vi "Test motor acceleration.vi"() -> ()   [LabVIEW 2016]
uses:
  <vilib>/Platform/TimedLoop/XDataNode/timing_clust.ctl
  <vilib>/Platform/TimedLoop/XDataNode/nitl_modes.ctl
  <vilib>/Platform/TimedLoop/XDataNode/wakeup.ctl
  <vilib>/Platform/TimedLoop/XDataNode/XDataNode.xnode
  <vilib>/Platform/TimedLoop/XDataNode/XDNodeRunTimeDep.lvlib
panel:
  in  "Disable motors":bool
  in  "Wheel velocity PID Right":T1={"P Gain"=0.8, "I Gain"=0.1, "D Gain"=0.002}
  in  "Wheel velocity PID Left":T1={"P Gain"=0.8, "I Gain"=0.1, "D Gain"=0.002}
  in  "Right motor speed rev/s":dbl
  in  "Left motor speed rev/s":dbl
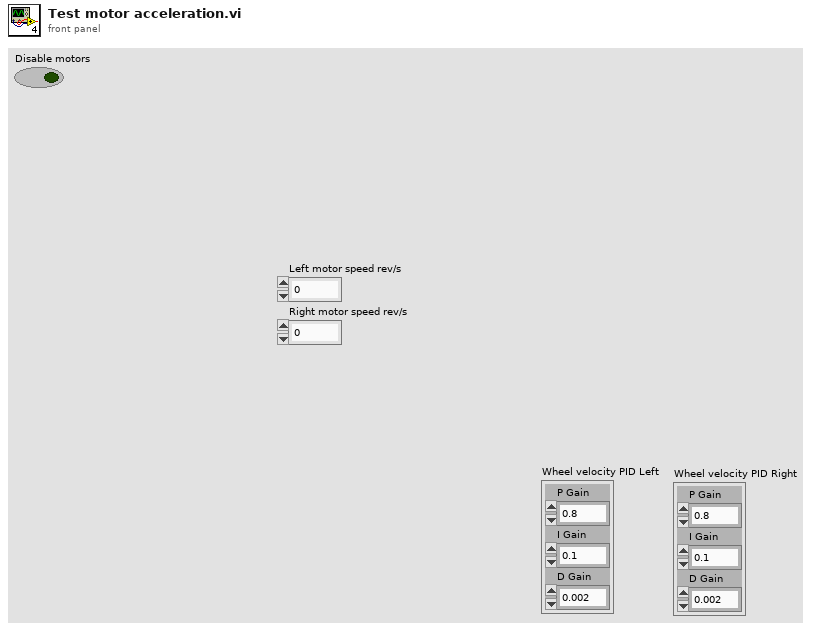
[diagram p1: front panel]
types:
  T1 = cluster{"P Gain":dbl, "I Gain":dbl, "D Gain":dbl}
  T2 = typedef "XDNodeRunTimeDep.lvlib/timing_clust.ctl" = cluster{"Expected End [f-1]":u64, "Actual End [f-1]":u64, "Finished Late? [f-1]":bool, "Expected End [i-1]":u64, "Actual End [i-1]":u64, "Finished Late? [i-1]":bool, "Expected Start [i]":u64, "Actual Start [i]":u64, "Expected Start [f]":u64, "Actual Start [f]":u64, "Source Name":string, "Structure Name":string, "Period":i64, "Deadline":i64, "Offset":i64, "Start":i64, "Priority":i32, "Timeout":i32, "Mode":T3, "Wakeup Reason":T4, "Error":errorcluster, "Source Type":string, "Secondary Source Type":string, "Global End Time":u64, "Global Start Time":u64, "Frame Duration":u64, "Iteration Duration":u64, "Assigned CPU":i32, "I/O Scan Engine Mode":u32}
  T3 = typedef "XDNodeRunTimeDep.lvlib/nitl_modes.ctl" = enum32{"No Change", "Process missed periods, maintain original phase", "Discard missed periods, maintain original phase", "Process missed periods, ignore original phase", "Discard missed periods, ignore original phase"}
  T4 = typedef "XDNodeRunTimeDep.lvlib/wakeup.ctl" = enum32{"Normal", "Aborted", "Asynchronous wakeup", "Timing source error", "Timed loop error", "Timeout"}
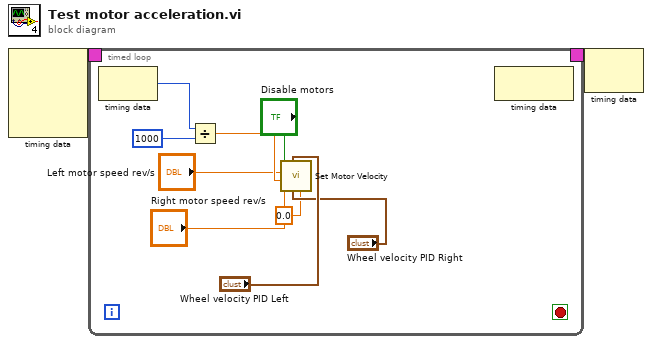
[diagram p0: block diagram]
diagram:
  n1 = node-c288() -> (w2:T2)  [unwired: 4 in]
  n2 = timed-loop {
    timing: w2 -> [_]
    timing-out: [_] -> w1
    stop <- _ stop-if-true
    n3 = node-c288() -> (w11:i64)  [unwired: 1 in]
    n4 = Divide(x=w11, y=i64 1000) -> (x/y=w9:dbl)
    n5 = call "Set Motor Velocity.vi"("Back motor speed rev/s"=0.0, "Motor Controller PID Gains Right"="Wheel velocity PID Right", "Motor Controller PID Gains Left"="Wheel velocity PID Left", "Disable motors"="Disable motors", "dt"=w9, "Right motor speed rev/s"="Right motor speed rev/s", "Left motor speed rev/s"="Left motor speed rev/s") -> ()  [unwired: 5 in]
    n6 = node-c288() -> ()  [unwired: 1 in, 1 out]
  }
  n7 = node-c288(w1) -> ()  [unwired: 1 out]
